vi "Write File.vi"(8 "error in (no error)":errorcluster, 11 "[User] Userinfo Binary in":refnum<class "[User] Userinfo Binary.lvclass">) -> (0 "error out":errorcluster, 3 "[User] Userinfo Binary out":refnum<class "[User] Userinfo Binary.lvclass">)   [LabVIEW 2020, in "[User] Userinfo Binary.lvclass"]
uses:
  [User] Userinfo Binary.lvclass
  [User] Userinfo Binary.lvclass/[User] Userinfo Binary.ctl
  <vilib>/YU/YU-Encrypt/AES/AES.lvclass
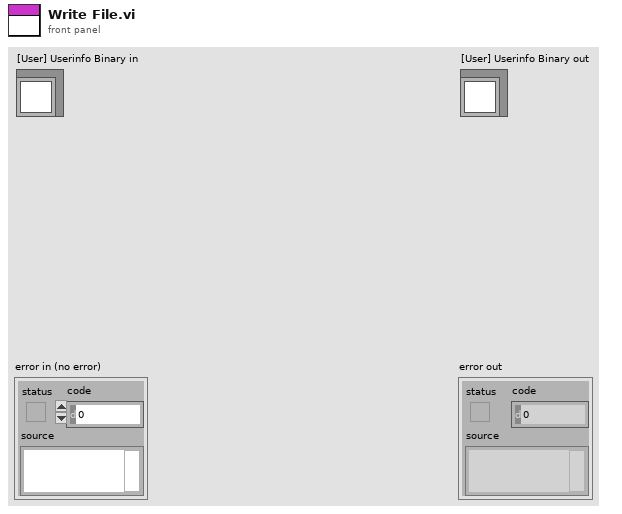
[diagram p1: front panel]
types:
  T1 = enum16{"open", "replace", "create", "open or create", "replace or create", "replace or create with confirmation"}
  T2 = typedef "[User] Userinfo Binary.lvclass/userinfo.ctl" = cluster{"password":string, "authority":i8, "department":string, "post":string, "remark":string, "create time":timestamp, "last login time":timestamp}
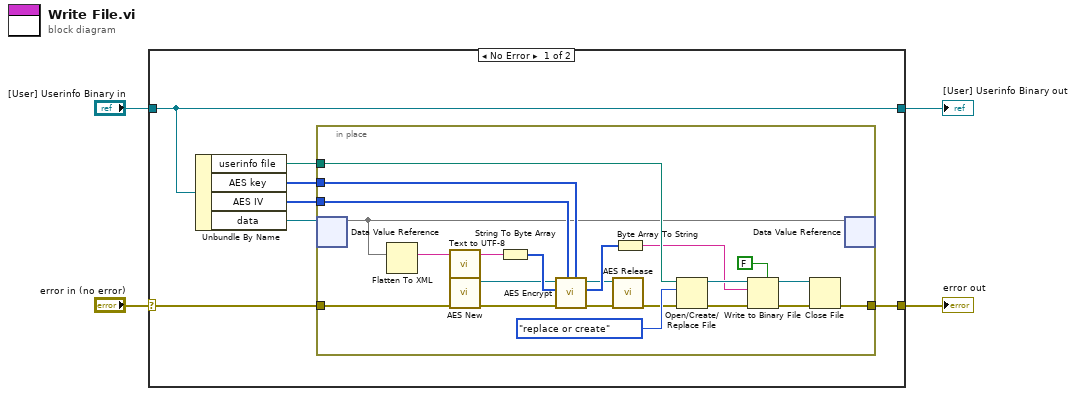
[diagram p0: block diagram]
diagram:
  n1 = case shown="No Error" "error in (no error)" {
    selector: "error in (no error)" -> [w5 w35]
    tunnel: [w7 w35] -> w1
    tunnel: [w11 w34] -> w2
    tunnel: "[User] Userinfo Binary in" -> [w11 w34]
    frame No Error {
      n2 = Unbundle By Name(w11) -> ("userinfo file"=w8:path, "AES key"=w10:u8[], "AES IV"=w9:u8[], "data"=w6:refnum<data-value>)
      n3 = in-place {
        in-place-border: w10 -> [w29]
        in-place-border: w9 -> [w28]
        in-place-border: w8 -> [w26]
        in-place-border: [w20] -> w7
        in-place-border: w5 -> [w14]
        n4 = in-place-dvr #1(w6) -> (w12:map{string, T2})  [unwired: 1 out]
        n5 = Flatten To XML(6:w12) -> (2:w13:string)
        n6 = call <vilib>:"Text to UTF-8.vi"("text"=w13) -> ("utf-8 text"=w32:string)  [unwired: 4 in]
        n7 = call <vilib>:"AES New.vi"("error in (no error)"=w14) -> ("error out"=w33:errorcluster, "AES out"=w30:refnum<class "AES.lvclass">)  [unwired: 9 in]
        n8 = String To Byte Array(string=w32) -> (unsigned byte array=w31:u8[])
        n9 = call <vilib>:"AES Encrypt.vi"("Key"=w29, "IV"=w28, "error in (no error)"=w33, "data"=w31, "AES in"=w30) -> ("error out"=w19:errorcluster, "encrypted data"=w27:u8[], "AES out"=w18:refnum<class "AES.lvclass">)  [unwired: 4 in]
        n10 = call <vilib>:"AES Release.vi"("error in (no error)"=w19, "AES in"=w18) -> ("error out"=w17:errorcluster)  [unwired: 9 in]
        n11 = Byte Array To String(unsigned byte array=w27) -> (string=w15:string)
        n12 = Open/Create/Replace File(file path (use dialog)=w26, error in=w17, operation (0:open)=T1."replace or create") -> (refnum out=w23:refnum<file>, error out=w24:errorcluster)  [unwired: 3 in, 1 out]
        n13 = Write to Binary File(file (use dialog)=w23, data=w15, error in=w24, 5:FALSE ("prepend array or string size? (T)")) -> (refnum out=w21:refnum<file>, error out=w22:errorcluster)  [unwired: 2 in, 1 out]
        n14 = Close File(refnum=w21, error in=w22) -> (error out=w20:errorcluster)  [unwired: 1 out]
        n15 = in-place-dvr #1(w12) -> ()  [unwired: 2 out]
      }
    }
    frame Error {
    }
  }
  "error out" <- w1
  "[User] Userinfo Binary out" <- w2
